vi "_QMH_Clear.vi"(8 "error in (no error)":errorcluster, 11 "QMH in":refnum<class "QMH.lvclass">) -> (0 "error out":errorcluster, 3 "QMH out":refnum<class "QMH.lvclass">)   [LabVIEW 2018, in "QMH.lvclass"]
uses:
  QMH.lvclass
  QMH.lvclass/QMH.ctl
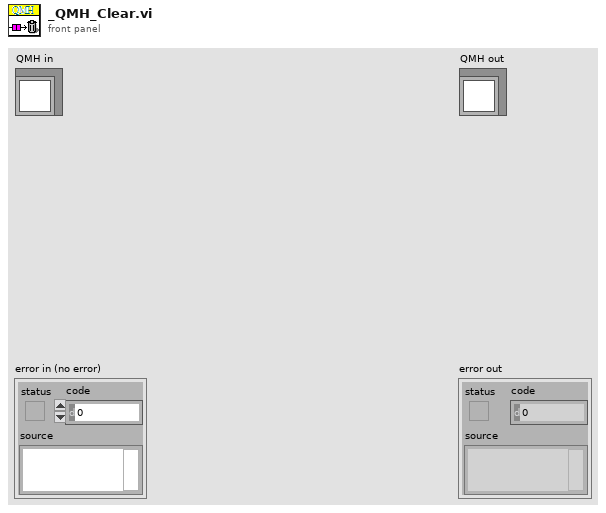
[diagram p1: front panel]
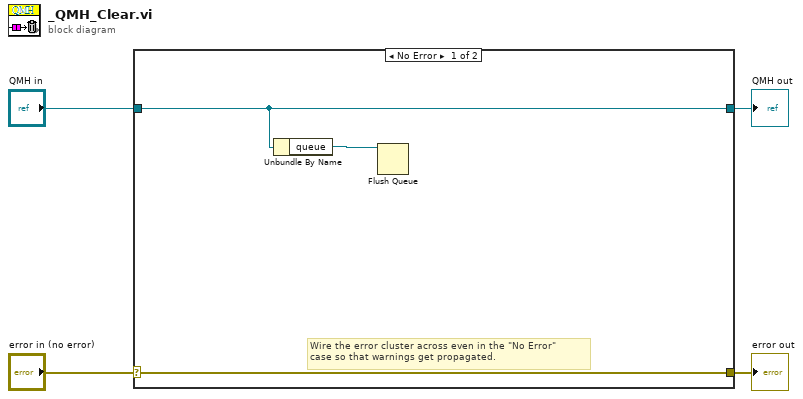
[diagram p0: block diagram]
diagram:
  n1 = case shown="No Error" "error in (no error)" {
    selector: "error in (no error)" -> [w7 w9]
    tunnel: [w7 w9] -> w3
    tunnel: [w6 w8] -> w1
    tunnel: "QMH in" -> [w6 w8]
    frame No Error {
      # "Wire the error cluster across even in the \"No Error\"\ncase so that warnings get propagated."
      n2 = Unbundle By Name(w6) -> ("queue"=w5:refnum<queue>)
      n3 = Flush Queue(queue=w5) -> ()  [unwired: 1 in, 3 out]
    }
    frame Error {
    }
  }
  "error out" <- w3
  "QMH out" <- w1
